vi "Test Instrument.vi"(7 "Unit Address (1)":i16=1, 8 "error in (no error)":errorcluster {"code" format="%.0x"}, 10 "Test Output (0: All Off)":i16(ring) items=["All Off", "Output 1A", "Output 1B", "Output 2A", "Output 2B", "Retransmit 1", "Retransmit 2", "Alarm 1", "Alarm 2", "Digital Output 1", "Digital Output 2", "Digital Output 3", "Digital Output 4", "Digital Output 5", "Digital Output 6", "Digital Output 7", "Digital Output 8", "All On", "Communications", "Display Test"], 11 "VISA resource name":refnum<visa-resource-name>) -> (0 "error out":errorcluster {"code" format="%.0x"}, 3 "VISA resource name out":refnum<visa-resource-name>)   [LabVIEW 2010]
doc: "This VI sets instrument outputs to testing state."
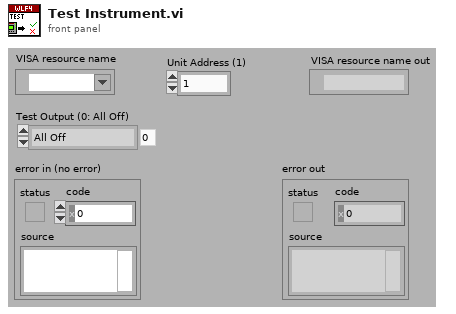
[diagram p1: front panel]
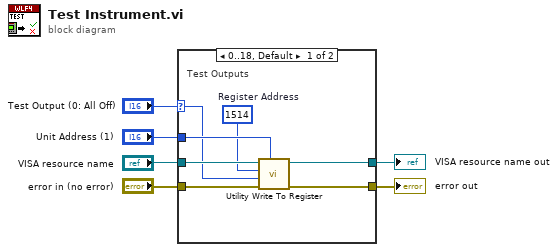
[diagram p0: block diagram]
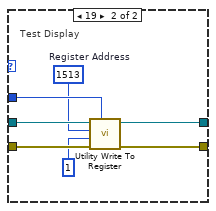
[diagram p2: hidden frame]
diagram:
  n1 = case shown="0..18, Default" "Test Output (0: All Off)" {
    selector: "Test Output (0: All Off)" -> [w7 _]
    tunnel: [w13 w20] -> w6
    tunnel: "Unit Address (1)" -> [w12 w19]
    tunnel: "VISA resource name" -> [w11 w18]
    tunnel: "error in (no error)" -> [w10 w17]
    tunnel: [w9 w16] -> w2
    frame 0..18, Default {
      w8 = u16 1514  # Register Address
      # "Test Outputs"
      n2 = call "Utility Write To Register.vi"("Unit Address (1)"=w12, "error in (no error)"=w10, "Data (0)"=w7, "Register Address (0)"=w8, "VISA resource name"=w11) -> ("error out"=w9:errorcluster, "VISA resource name out"=w13:refnum<visa-resource-name>)  [unwired: 5 in]
    }
    frame 19 {
      w15 = u16 1513  # Register Address
      # "Test Display"
      n3 = call "Utility Write To Register.vi"("Unit Address (1)"=w19, "error in (no error)"=w17, "Data (0)"=i16 1, "Register Address (0)"=w15, "VISA resource name"=w18) -> ("error out"=w16:errorcluster, "VISA resource name out"=w20:refnum<visa-resource-name>)  [unwired: 5 in]
    }
  }
  "error out" <- w2
  "VISA resource name out" <- w6
